vi "Genealogy.vi"(0 "Barcode":string, 7 "SessionID":string, 11 "Error In":errorcluster) -> (4 "Pass":bool, 15 "Error Out":errorcluster)   [LabVIEW 2021]
doc: "Takes a scanned barcode, breaks it down to PN and SN, writes it using UDS and confrims the genealogy by reading it back."
uses:
  Lunar Libraries/UDS CAN/Controls/UDSGenealogyItems.ctl
  <vilib>/regexp/Match Regular Expression.xnode
  Lunar Libraries/UDS CAN/Lunar UDS CAN.lvlib
panel:
  # "Inputs"
  # "Outputs"
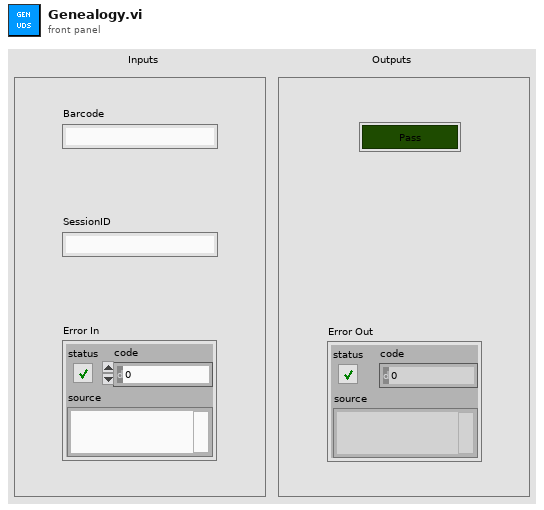
[diagram p1: front panel]
types:
  T1 = typedef "Lunar UDS CAN.lvlib/UDSGenealogyItems.ctl" = enum16{"AppHeader", "Genealogy Block Init", "Genealogy Block", "Board Part Number", "Board Serial Number", "Aux1 Part Number", "Aux1 Serial Number", "Aux2 Part Number", "Aux2 Serial Number", "Config Block Init", "Config Block", "Calibration Block Init", "Calibration Block", "Node Data Block Init", "Node Data Block", "Can Bus Instance"}
  T2 = typedef "Lunar UDS CAN.lvlib/UDSReadData.ctl" = cluster{"DataString":string, "Data":i32[]}
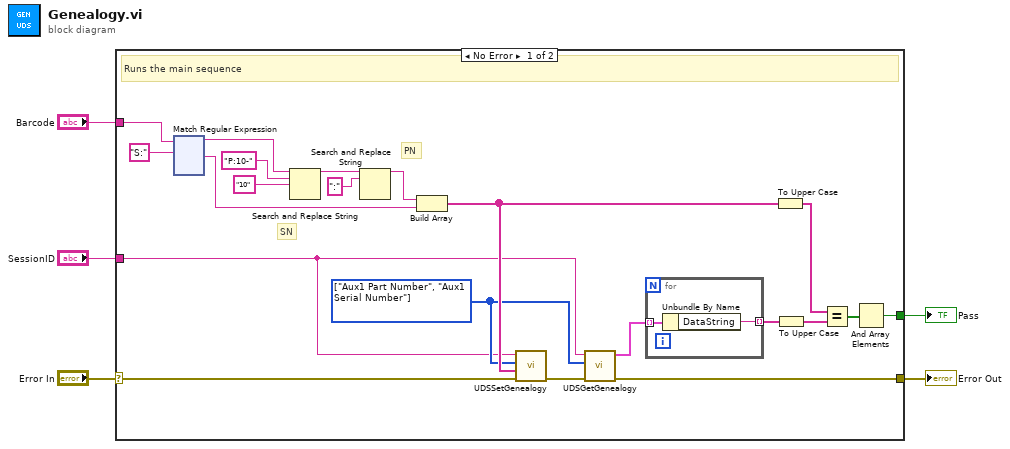
[diagram p0: block diagram]
diagram:
  n1 = case shown="No Error" "Error In" {
    selector: "Error In" -> [w16 w146]
    tunnel: "Barcode" -> [w26 _]
    tunnel: [w14 w146] -> w3
    tunnel: [w8 _] -> w2
    tunnel: "SessionID" -> [w6 _]
    frame No Error {
      w7 = T1[] [enum."Aux1 Part Number", enum."Aux1 Serial Number"] items=["AppHeader", "Genealogy Block Init", "Genealogy Block", "Board Part Number", "Board Serial Number", "Aux1 Part Number", "Aux1 Serial Number", "Aux2 Part Number", "Aux2 Serial Number", "Config Block Init", "Config Block", "Calibration Block Init", "Calibration Block", "Node Data Block Init", "Node Data Block", "Can Bus Instance"] ("GenealogyItemsToSet")
      # "SN"
      # "PN"
      # "Runs the main sequence"
      n2 = xnode "Match Regular Expression"("input string"=w26, "regular expression"="S:") -> ("before match"=w23:string, "after match"=w17:string)  [unwired: 4 in, 3 out]
      n3 = Search and Replace String(input string=w23, search string="P:10-", replace string="10" ("search string")) -> (result string=w24:string)  [unwired: 5 in, 3 out]
      n4 = Search and Replace String(input string=w24, search string=":") -> (result string=w18:string)  [unwired: 6 in, 3 out]
      n5 = Build Array(w18, w17) -> (w12:string[])
      n6 = call "UDSSetGenealogy.vi"("Error In"=w16, "DataToSet"=w12, "GenealogyItemsToSet"=w7, "SessionID"=w6) -> ("Error Out"=w25:errorcluster)  [unwired: 6 in, 1 out]
      n7 = call "UDSGetGenealogy.vi"("error in (no error)"=w25, "GenealogyItemsToRead"=w7, "SessionID"=w6) -> ("error Out"=w14:errorcluster, "ReadGenealogyData"=w15:T2[])  [unwired: 6 in, 1 out]
      n8 = for {
        tunnel: w15 -> [w28] mode=indexing
        tunnel: [w27] -> w13 mode=indexing
        n9 = Unbundle By Name(w28) -> ("DataString"=w27:string)
      }
      n10 = To Upper Case(1:w12) -> (0:w10:string[])
      n11 = To Upper Case(1:w13) -> (0:w11:string[])
      n12 = Equal?(x=w10, y=w11) -> (x = y?=w9:bool[])
      n13 = And Array Elements(Boolean array=w9) -> (logical AND=w8:bool)
    }
    frame Error {
      # "Can't start due to error"
    }
  }
  "Error Out" <- w3
  "Pass" <- w2
